vi "Empirical Mode Decomposition.vi"(7 "IMF Tolerance":dbl=0.2 format="%#_13g", 11 "Waveform":waveform(dbl)) -> (0 "df":dbl, 1 "dt":dbl, 2 "Hilbert Spectra":dbl[][][](array[numeric]), 3 "IMF Array":waveform(dbl)[](array[waveform]))   [LabVIEW 2013, in "Empirical Mode Decomposition.lvlib"]
uses:
  <vilib>/Analysis/4window.llb/windowTd.ctl
  <vilib>/Analysis/8numeric.llb/1D Numeric Integration.vi
  <vilib>/Waveform/WDTOps.llb/WDT Waveform Duration DBL.vi
  <vilib>/measure/maspectr.llb/FFT Spectrum (Mag-Phase) for 1 Chan.vi
  <vilib>/measure/maspectr.llb/FFT Power Spectrum and PSD for 1 Chan.vi
  Empirical Mode Decomposition.lvlib
  <vilib>/measure/NI_MAPro.lvlib
  <vilib>/Analysis/NI_AALPro.lvlib
  <vilib>/Analysis/NI_AAL_SigProc.lvlib
  <vilib>/gmath/NI_Gmath.lvlib
panel:
  out "Signal":waveform(dbl)(graph)
  out "Null Integral":i32[](graph)
  out "Degree of Stationarity":dbl[](graph)
  out "Instantaneous Energy Density Level":dbl[](graph)
  out "Marginal Hilbert Spectrum":dbl[](graph)
  out "Hilbert Spectrum":dbl[][](graph)
  out "IMF":waveform(dbl)(graph)
  out "Waveform Graph":cluster{"f0":dbl, "df":dbl, "magnitude":dbl[]}(graph)
  out "error":i32
  out "size(s)":i32
  in  "Max Iterations":i32=1000
  out "IMF Index":i32
  out "ci Spectrum":cluster{"f0":dbl, "df":dbl, "magnitude":dbl[]}[](graph)
  out "Residual":waveform(dbl)(graph)
  # "TODO: Smooth out the Hilbert Spectrum graph"
  # "Scale                  Index\n1                              512-1023\n2                              256-511\n3                              128-255\n4                              64-127\n5                              32-63\n6                              16-31\n7                              8-15\n8                              4-7\n9                              2-3"
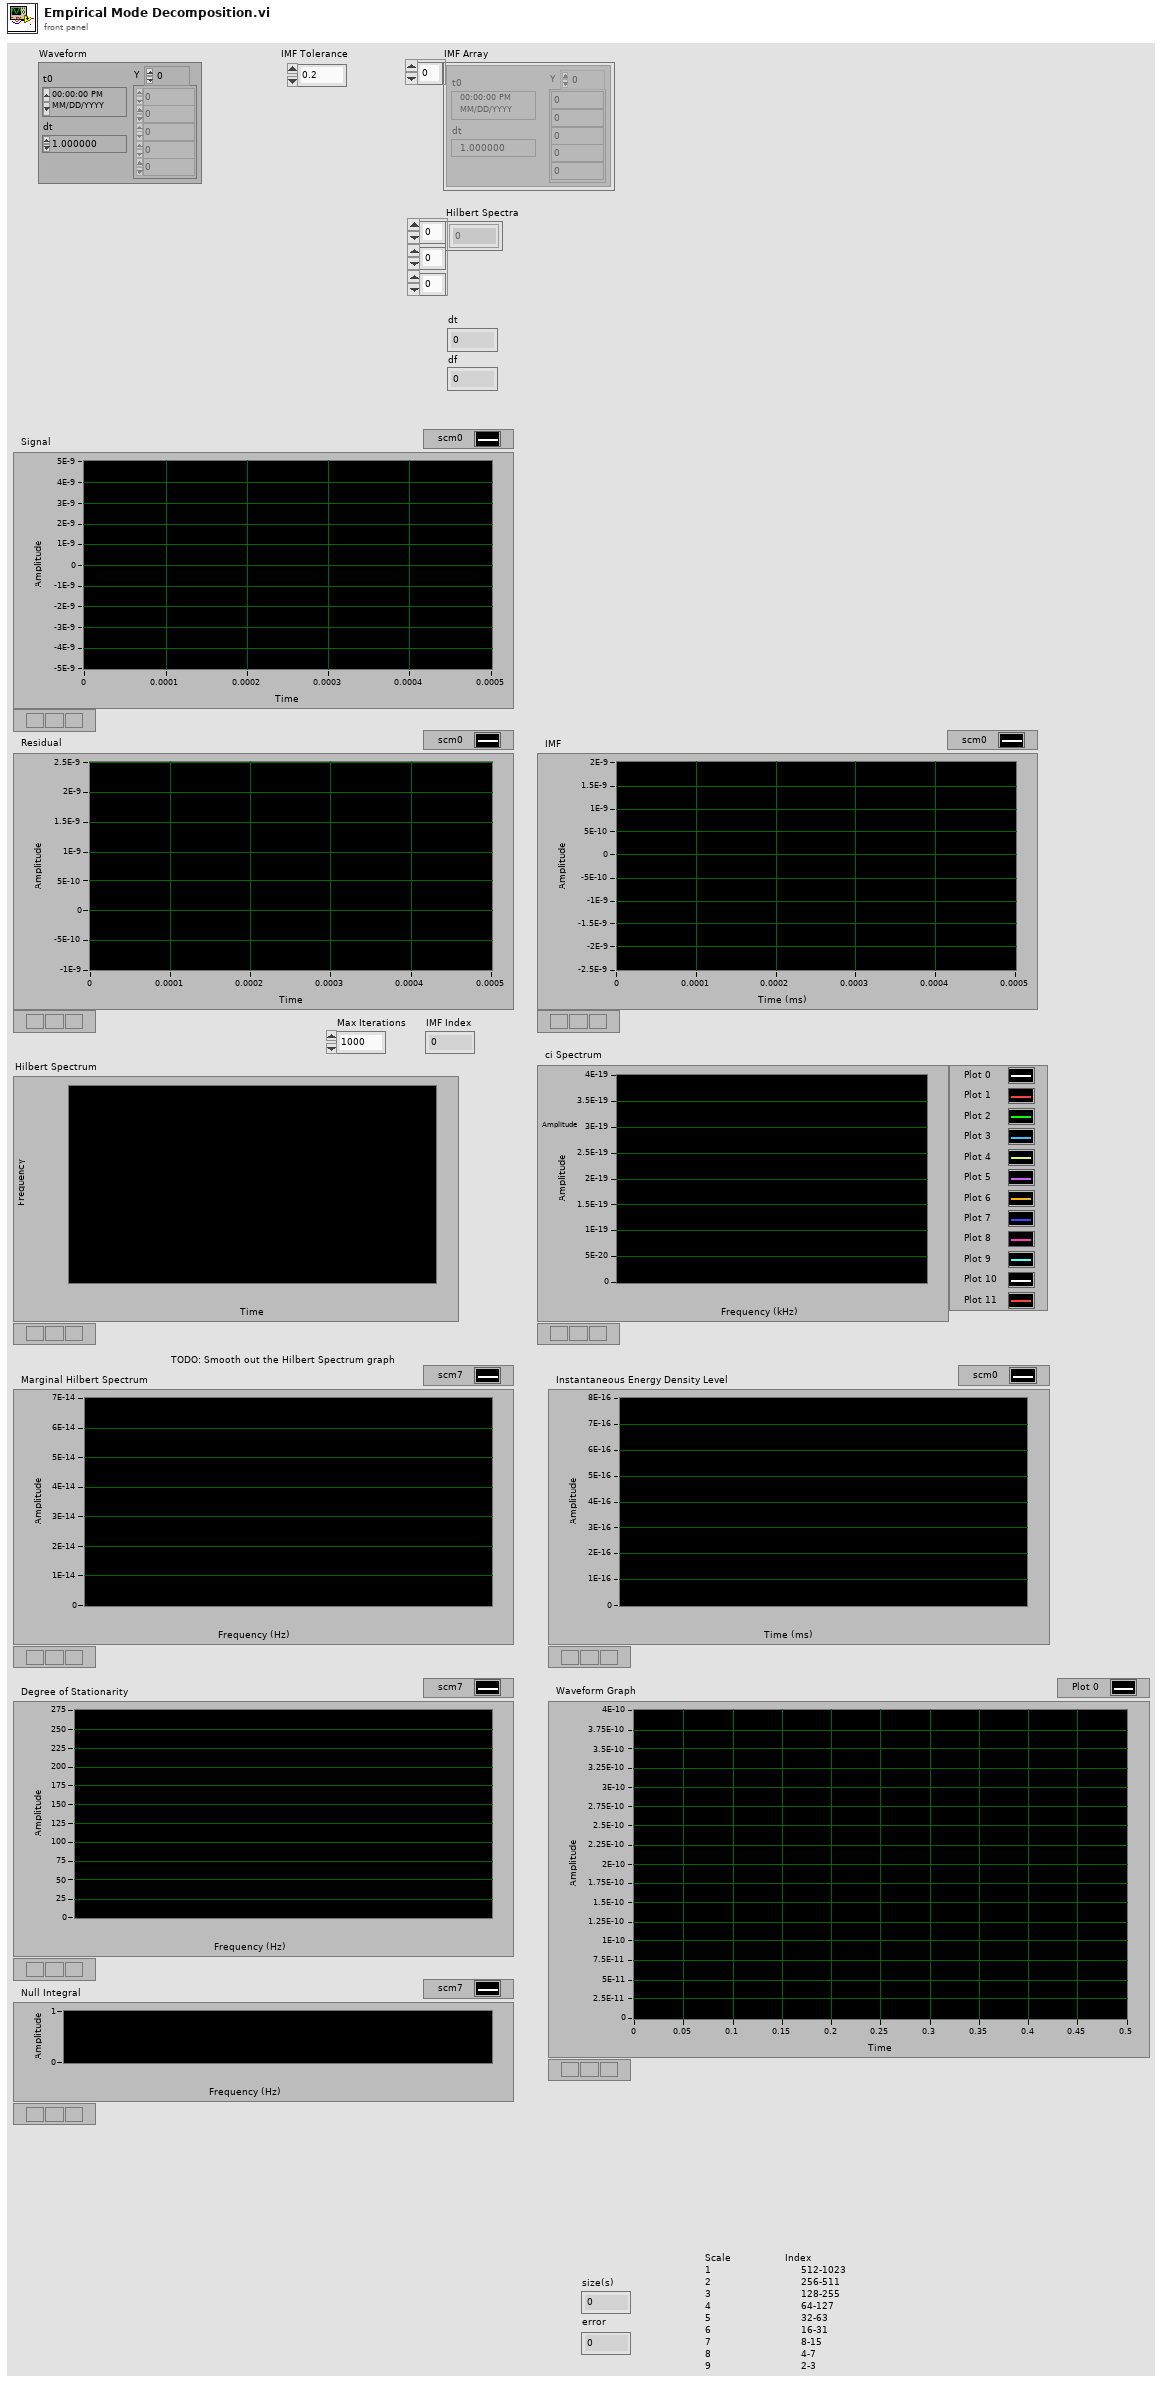
[diagram p1: front panel]
types:
  T1 = typedef "NI_AALPro.lvlib/windowTd.ctl" = u32
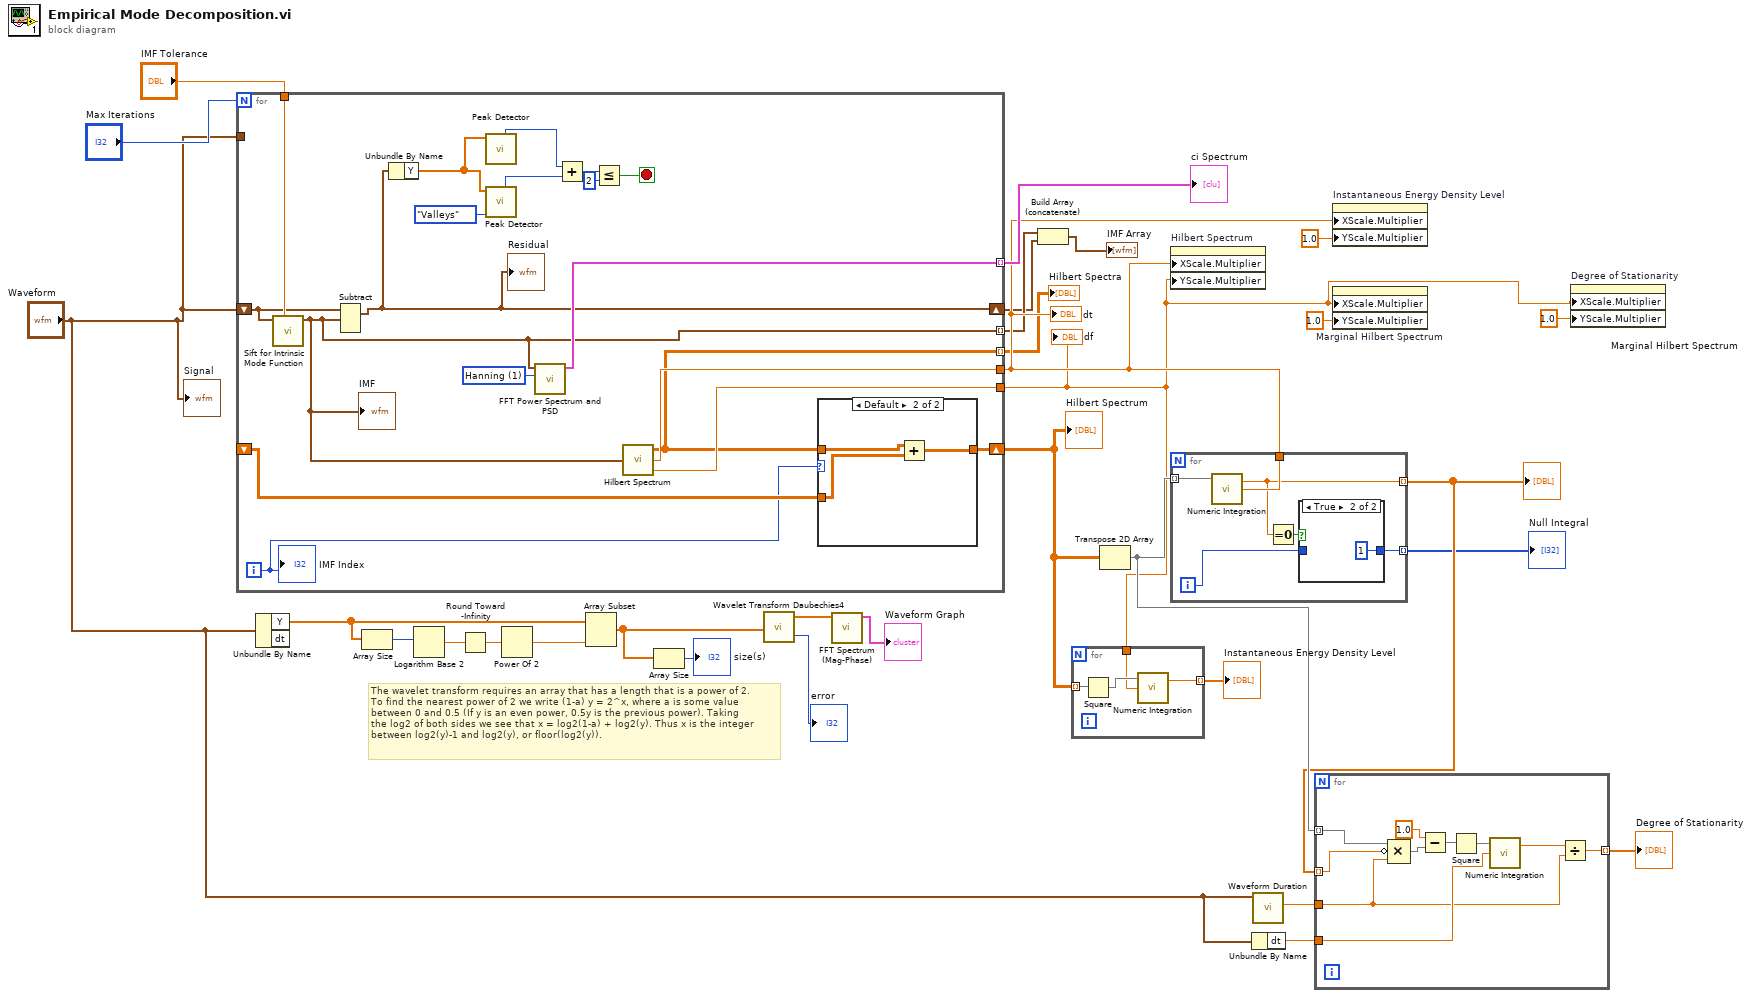
[diagram p0: block diagram]
diagram:
  # "The wavelet transform requires an array that has a length that is a power of 2.\nTo find the nearest power of 2 we write (1-a) y = 2^x, where a is some value\nbetween 0 and 0.5 (If y is an even power, 0.5y is the previous power). Taking\nthe log2 of both sides we see that x = log2(1-a) + log2(y). Thus x is the integer\nbetween log2(y)-1 and log2(y), or floor(log2(y))."
  n1 = for {
    N: "Max Iterations" -> [_]
    tunnel: "IMF Tolerance" -> [w50]
    shift-right: [w32] -> w3
    shift-left: "Waveform" -> [w49]
    tunnel: [w39] -> w4 mode=indexing
    tunnel: "Waveform" -> [_]
    tunnel: [w46] -> w29 mode=indexing
    shift-right: [w38] -> w9
    shift-left: _ -> [w37]
    tunnel: [w36] -> w11
    tunnel: [w35] -> w8
    tunnel: [w33] -> w5 mode=indexing
    i -> [w34]
    stop <- w48 stop-if-true
    w47 = T1 1 items=["Rectangle"=0, "Hanning"=1, "Hamming"=2, "Blackman-Harris"=3, "Exact Blackman"=4, "Blackman"=5, "Flat Top"=6, "4 Term B-Harris "=7, "7 Term B-Harris"=8, "Low Sidelobe"=9, "Blackman Nuttall"=11, "Triangle"=30, "Bartlett-Hanning"=31, "Bohman"=32, "Parzen"=33, "Welch"=34, "Kaiser"=60, "Dolph-Chebyshev"=61, "Gaussian"=62] ("window")
    n2 = call "Sift for Intrinsic Mode Function.vi"("Tolerance (1e-9)"=w50, "Waveform"=w49) -> ("IMF"=w39:waveform(dbl))  [unwired: 9 in]
    "IMF" <- w39
    n3 = Subtract(1:w39, 2:w49) -> (0:w32:waveform(dbl))  [unwired: 1 in, 1 out]
    "Residual" <- w32
    n4 = Unbundle By Name(w32) -> ("Y"=w45:dbl[])
    n5 = call <vilib>:"Peak Detector.vi"("X"=w45) -> ("# found"=w43:i32)  [unwired: 6 in, 4 out]
    n6 = call <vilib>:"Peak Detector.vi"("peaks/valleys"=enum32{"Peaks", "Valleys"}."Valleys", "X"=w45) -> ("# found"=w42:i32)  [unwired: 5 in, 4 out]
    n7 = call-poly <vilib>:"FFT Power Spectrum and PSD.vi"("window"=w47, "time signal"=w39) -> ("Power Spectrum / PSD"=w46:cluster{"f0":dbl, "df":dbl, "magnitude":dbl[]})  [unwired: 6 in, 3 out]
    n8 = Add(x=w43, y=w42) -> (x+y=w41:i32)
    n9 = Less Or Equal?(x=w41, y=2) -> (x <= y?=w48:bool)
    n10 = call "Hilbert Spectrum.vi"("Waveform"=w39) -> ("df"=w35:dbl, "dt"=w36:dbl, "Spectrum"=w33:dbl[][])  [unwired: 2 in]
    n11 = case shown="Default" w34 {
      tunnel: w33 -> [w51 w53]
      tunnel: [w51 w54] -> w38
      tunnel: w37 -> [_ w52]
      frame 0 {
      }
      frame Default {
        n12 = Add(x=w53, y=w52) -> (x+y=w54:dbl[][])
      }
    }
    "IMF Index" <- w34
  }
  "ci Spectrum" <- w29
  "Hilbert Spectrum" <- w9
  "Hilbert Spectra" <- w5
  "dt" <- w11
  "df" <- w8
  n13 = Unbundle By Name("Waveform") -> ("Y"=w28:dbl[])  [unwired: 1 out]
  n14 = Array Size(array=w28) -> (size(s)=w25:i32)
  n15 = Logarithm Base 2(1:w25) -> (0:w23:dbl)
  n16 = Round Toward -Infinity(1:w23) -> (0:w24:dbl)
  n17 = Power Of 2(x=w24) -> (2^x=w22:dbl)
  n18 = Array Subset(array=w28, length=w22) -> (w27:dbl[])  [unwired: 1 in]
  n19 = Array Size(array=w27) -> (size(s)=→"size(s)":i32)
  n20 = call <vilib>:"Wavelet Transform Daubechies4.vi"("X"=w27) -> ("Wavelet Daubechies4 {X}"=w20:dbl[], "error"=→"error":i32)
  n21 = call-poly <vilib>:"FFT Spectrum (Mag-Phase).vi"("time signal"=w20) -> ("magnitude"=→"Waveform Graph":cluster{"f0":dbl, "df":dbl, "magnitude":dbl[]})  [unwired: 6 in, 4 out]
  n22 = Build Array (concatenate)(w4, w3) -> (→"IMF Array":waveform(dbl)[])
  n23 = for {
    tunnel: w9 -> [w58] mode=indexing
    tunnel: w8 -> [w56]
    tunnel: [w55] -> w7 mode=indexing
    n24 = Square(x=w58) -> (x^2=w57:dbl[])
    n25 = call-poly <vilib>:"Numeric Integration.vi"("dt"=w56, "Input Array"=w57) -> ("result"=w55:dbl)  [unwired: 1 in, 1 out]
  }
  "Instantaneous Energy Density Level" <- w7
  n26 = Transpose 2D Array(2D array=w9) -> (transposed array=w12:dbl[][])
  n27 = property on="Hilbert Spectrum" class="IntGraph (strict)"("XScale.Multiplier"=w11, "YScale.Multiplier"=w8) -> ()  [unwired: 2 in, 2 out]
  n28 = for {
    tunnel: w12 -> [w64] mode=indexing
    tunnel: w11 -> [w63]
    tunnel: [w61] -> w10 mode=indexing
    tunnel: [w59] -> w6 mode=indexing
    i -> [w60]
    n29 = call-poly <vilib>:"Numeric Integration.vi"("dt"=w63, "Input Array"=w64) -> ("result"=w61:dbl)  [unwired: 1 in, 1 out]
    n30 = Equal To 0?(x=w61) -> (x = 0?=w62:bool)
    n31 = case shown="True" w62 {
      tunnel: w60 -> [_ _]
      tunnel: [_ 1] -> w59
      frame False {
      }
      frame True {
      }
    }
  }
  "Marginal Hilbert Spectrum" <- w10
  "Null Integral" <- w6
  n32 = Unbundle By Name("Waveform") -> ("dt"=w15:dbl)
  n33 = call-poly <vilib>:"Waveform Duration.vi"("waveform in"="Waveform") -> ("duration"=w16:dbl)  [unwired: 8 in, 2 out]
  n34 = for {
    tunnel: w12 -> [w75] mode=indexing
    tunnel: w10 -> [w70] mode=indexing
    tunnel: w16 -> [w72]
    tunnel: w15 -> [w74]
    tunnel: [w71] -> w14 mode=indexing
    n35 = Compound Arithmetic op=MULTIPLY(w75, invert w70, w72) -> (w69:dbl[])
    n36 = Subtract(x=1.0, y=w69) -> (x-y=w67:dbl[])
    n37 = Square(x=w67) -> (x^2=w66:dbl[])
    n38 = call-poly <vilib>:"Numeric Integration.vi"("dt"=w74, "Input Array"=w66) -> ("result"=w73:dbl)  [unwired: 1 in, 1 out]
    n39 = Divide(x=w73, y=w72) -> (x/y=w71:dbl)
  }
  "Degree of Stationarity" <- w14
  n40 = property on="Instantaneous Energy Density Level" class="WFGraph (strict)"("XScale.Multiplier"=w11, "YScale.Multiplier"=1.0 ("Y Scale.Offset and Multiplier:Multiplier")) -> ()  [unwired: 2 in, 2 out]
  n41 = property on="Marginal Hilbert Spectrum" class="WFGraph (strict)"("XScale.Multiplier"=w8, "YScale.Multiplier"=1.0 ("Y Scale.Offset and Multiplier:Multiplier")) -> ()  [unwired: 2 in, 2 out]
  n42 = property on="Degree of Stationarity" class="WFGraph (strict)"("XScale.Multiplier"=w8, "YScale.Multiplier"=1.0 ("Y Scale.Offset and Multiplier:Multiplier")) -> ()  [unwired: 2 in, 2 out]
  "Signal" <- "Waveform"
